vi "自然数平方和.vi"(11 "范围":i32=100) -> (3 "和":i32)   [LabVIEW 2012]
doc: "功能：\n\n求自然数的平方和。\n\n公式：\n\nSn=1^2+2^....+n^2\n\ncsxcs_366创建"
panel:
  out "验证":bool
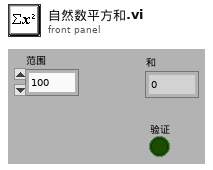
[diagram p1: front panel]
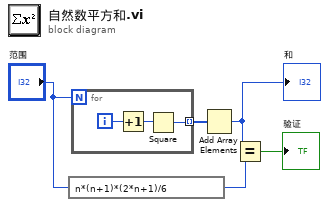
[diagram p0: block diagram]
diagram:
  n1 = expression code="n*(n+1)*(2*n+1)/6"("范围") -> (w2:i32)
  n2 = for {
    N: "范围" -> [_]
    tunnel: [w6] -> w5 mode=indexing
    i -> [w8]
    n3 = Increment(x=w8) -> (x+1=w7:i32)
    n4 = Square(x=w7) -> (x^2=w6:i32)
  }
  n5 = Add Array Elements(numeric array=w5) -> (sum=w3:i32)
  "和" <- w3
  n6 = Equal?(x=w3, y=w2) -> (x = y?=→"验证":bool)
